vi "Compile Communication Configuration.vi"(8 "error in (no error)":errorcluster, 11 "Device Ref in":T1 format="%.0x") -> (0 "error out":errorcluster, 2 "Communication Configuration":T2, 3 "Device Ref out":T1 format="%.0x")   [LabVIEW 2017, in "Routing and Faulting System Explorer.lvlib"]
uses:
  Routing and Faulting System Explorer.lvlib
  Shared/Communication Configuration.ctl
  <vilib>/NI Veristand/Custom Device API/Custom Device Item Ref.ctl
  Shared/Routing and Faulting Shared.lvlib
  <vilib>/NI Veristand/Custom Device API/Custom Device API.lvlib
  Shared/Routing and Faulting Consumer System Definition API/Routing and Faulting Hardware API.lvlib
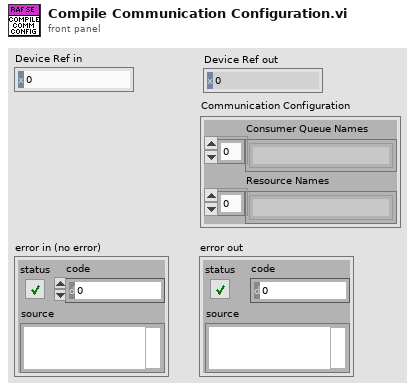
[diagram p1: front panel]
types:
  T1 = typedef "Custom Device API.lvlib/Custom Device Item Ref.ctl" = u64
  T2 = typedef "Routing and Faulting Shared.lvlib/Communication Configuration.ctl" = cluster{"Consumer Queue Names":string[], "Resource Names":string[]}
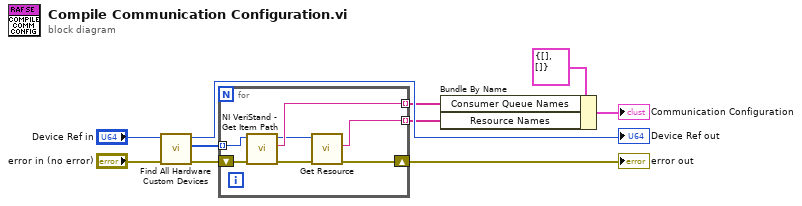
[diagram p0: block diagram]
diagram:
  n1 = call "Find All Hardware Custom Devices.vi"("error in (no error)"="error in (no error)", "Routing and Faulting Ref in"="Device Ref in") -> ("error out"=w6:errorcluster, "Hardware Refs"=w3:T1[], "Routing and Faulting Ref out"=→"Device Ref out":T1)  [unwired: 7 in]
  n2 = for {
    shift-right: [w13] -> w5
    shift-left: w6 -> [w16]
    tunnel: w3 -> [w15] mode=indexing
    tunnel: [w17] -> w2 mode=indexing
    tunnel: [w11] -> w1 mode=indexing
    n3 = call <vilib>:"NI VeriStand - Get Item Path.vi"("error in (no error)"=w16, "Item Ref in"=w15) -> ("error out"=w14:errorcluster, "Path"=w17:string, "Item Ref out"=w12:T1)  [unwired: 6 in, 1 out]
    n4 = call "Get Resource.vi"("error in (no error)"=w14, "Hardware Ref in"=w12) -> ("error out"=w13:errorcluster, "Resource"=w11:string)  [unwired: 7 in, 1 out]
  }
  "error out" <- w5
  n5 = Bundle By Name(cluster=T2 {"Consumer Queue Names"=[], "Resource Names"=[]} ("Communication Configuration 2"), "Consumer Queue Names"=w2, "Resource Names"=w1) -> (→"Communication Configuration":T2)
